vi "ModifyWaveCTRLLocation.vi"(11 "队列输入":refnum<queue>) -> ()   [LabVIEW 2012, in "WaveGraphX.xctl"]
uses:
  WaveGraphX.xctl
  <vilib>/Utility/miscctls.llb/LVPoint32TypeDef.ctl
panel:
  in  "波形图":refnum<vi>
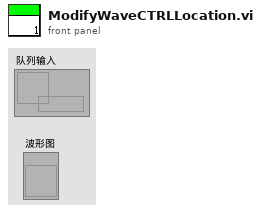
[diagram p1: front panel]
types:
  T1 = typedef "LVPoint32TypeDef.ctl" = cluster{"Horizontal":i32, "Vertical":i32}
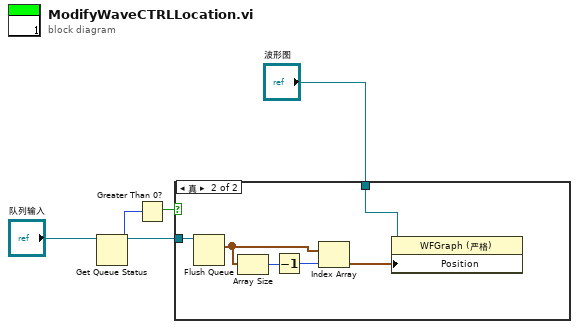
[diagram p0: block diagram]
diagram:
  n1 = Get Queue Status(queue="队列输入") -> (queue out=w5:refnum<queue>, # elements in queue=w3:i32)  [unwired: 2 in, 6 out]
  n2 = Greater Than 0?(x=w3) -> (x > 0?=w4:bool)
  n3 = case shown="真" w4 {
    tunnel: w5 -> [_ w11]
    tunnel: "波形图" -> [_ w6]
    frame False {
    }
    frame True {
      n4 = Flush Queue(queue=w11) -> (remaining elements=w9:T1[])  [unwired: 1 in, 2 out]
      n5 = Array Size(array=w9) -> (size(s)=w10:i32)
      n6 = Decrement(x=w10) -> (x-1=w8:i32)
      n7 = Index Array(array=w9, index=w8) -> (element=w7:T1)
      n8 = property class="WFGraph (严格)"(reference=w6, "Position"=w7) -> ()  [unwired: 1 in, 2 out]
    }
  }
